vi "Drive_AutoShift (1).vi"(5 "Max":dbl format="%#_13g", 6 "Force Low Gear":bool, 7 "ShifterRef":T2={"DevStatus"={"status"=FALSE, "code"=0, "source"=""}, "Pneumatics Control Module"=0, "Forward Solenoid Channel"=enum."Invalid", "Reverse Solenoid Channel"=enum."Invalid"}, 8 "Right  Input":dbl, 9 "Left Input":dbl, 10 "Right RPM":dbl, 11 "Left RPM":dbl) -> (1 "Shifting":bool, 2 "Right Output":dbl, 3 "Left Output":dbl, 4 "Gear":T1)   [LabVIEW 2017]
uses:
  <vilib>/Rock Robotics/WPI/Solenoid/WPI_SolenoidDevRef.ctl
  <vilib>/Rock Robotics/WPI/Solenoid/WPI_SolenoidChannel.ctl
  <vilib>/Rock Robotics/WPI/Solenoid/WPI_SolenoidValue.ctl
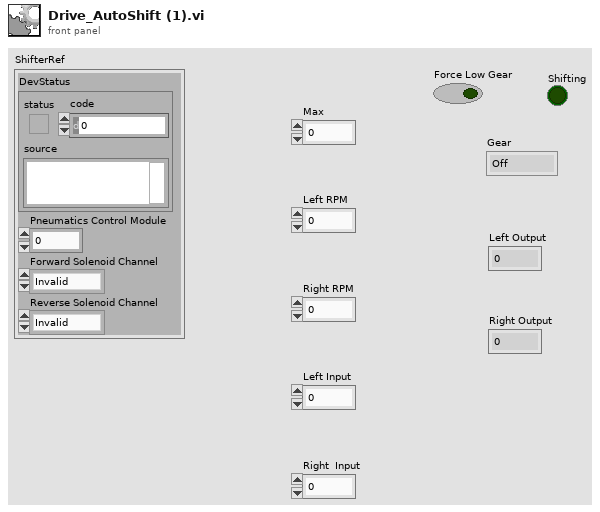
[diagram p1: front panel]
types:
  T1 = typedef "WPI_SolenoidValue.ctl" = enum16{"Off", "On", "Forward", "Reverse"}
  T2 = typedef "WPI_SolenoidDevRef.ctl" = cluster{"DevStatus":errorcluster, "Pneumatics Control Module":u8, "Forward Solenoid Channel":T3, "Reverse Solenoid Channel":T3}
  T3 = typedef "WPI_SolenoidChannel.ctl" = enum8{"Solenoid 0", "Solenoid 1", "Solenoid 2", "Solenoid 3", "Solenoid 4", "Solenoid 5", "Solenoid 6", "Solenoid 7", "Invalid"}
  T4 = cluster{"OutputMAX":dbl, "OutputMIN":dbl, "InputMAX":dbl, "InputMIN":dbl}
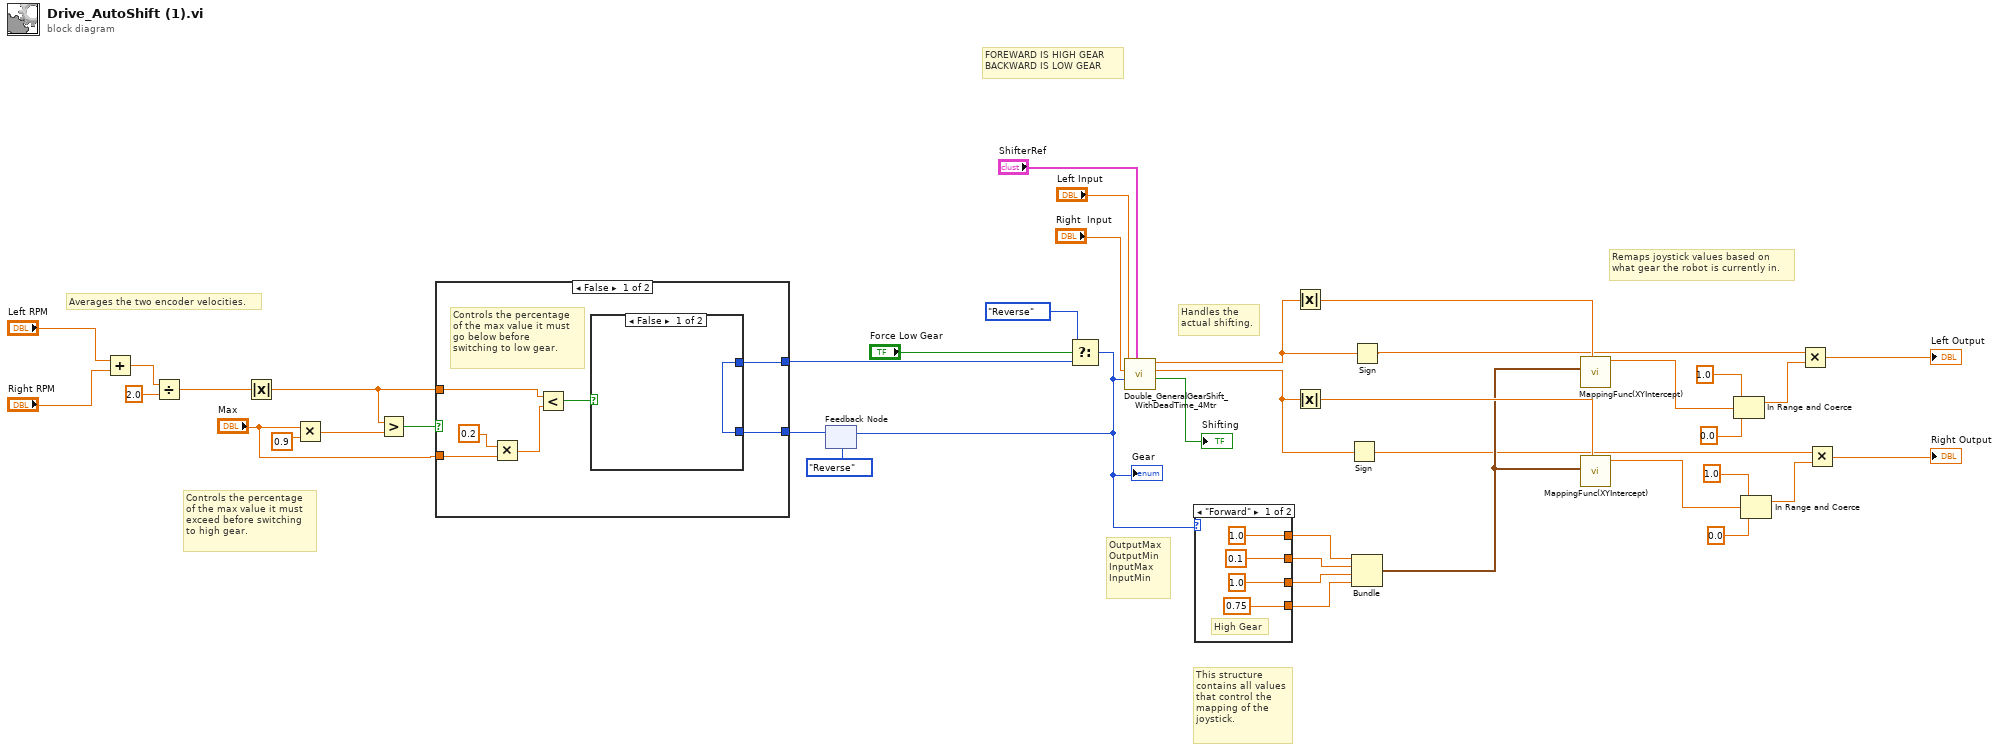
[diagram p0: block diagram]
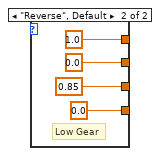
[diagram p2: hidden frame]
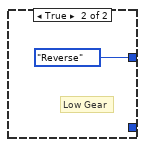
[diagram p3: hidden frame]
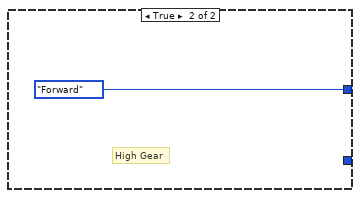
[diagram p4: hidden frame]
diagram:
  # "OutputMax\nOutputMin\nInputMax\nInputMin"
  # "This structure\ncontains all values\nthat control the\nmapping of the \njoystick."
  # "Remaps joystick values based on\nwhat gear the robot is currently in."
  # "Handles the\nactual shifting."
  # "FOREWARD IS HIGH GEAR\nBACKWARD IS LOW GEAR"
  # "Controls the percentage\nof the max value it must \nexceed before switching\nto high gear."
  # "Averages the two encoder velocities."
  n1 = Add(x="Left RPM", y="Right RPM") -> (x+y=w32:dbl)
  n2 = Divide(x=w32, y=2.0) -> (x/y=w12:dbl)
  n3 = Absolute Value(x=w12) -> (abs(x)=w11:dbl)
  n4 = Multiply(x="Max", y=0.9) -> (x*y=w40:dbl)
  n5 = Greater?(x=w11, y=w40) -> (0:w39:bool)
  n6 = feedback #1(WPI_SolenoidValue."Reverse" ("Shift Value")) -> (w9:T1)
  n7 = case shown="False" w39 {
    tunnel: [w44 WPI_SolenoidValue."Forward" ("Shift Value")] -> w23
    tunnel: "Max" -> [w47 _]
    tunnel: w9 -> [w43 _]
    tunnel: w11 -> [w42 _]
    frame False {
      # "Controls the percentage\nof the max value it must \ngo below before \nswitching to low gear."
      n8 = Multiply(x=0.2, y=w47) -> (x*y=w45:dbl)
      n9 = Less?(x=w42, y=w45) -> (x < y?=w48:bool)
      n10 = case shown="False" w48 {
        tunnel: [w49 WPI_SolenoidValue."Reverse" ("Shift Value")] -> w44
        tunnel: w43 -> [w49 _]
        frame False {
        }
        frame True {
          # "Low Gear"
        }
      }
    }
    frame True {
      # "High Gear"
    }
  }
  n11 = Select(t=WPI_SolenoidValue."Reverse", s="Force Low Gear", f=w23) -> (s? t:f=w1:T1)
  "Gear" <- w1
  n12 = feedback-in #1(w1) -> ()
  n13 = call "Double_GeneralGearShift_WithDeadTime_4Mtr.vi"("ShifterRef"="ShifterRef", "Shift Value"=w1, "Right"="Right  Input", "Left"="Left Input") -> ("Shifting"=→"Shifting":bool, "Right Output"=w6:dbl, "Left Output"=w7:dbl)  [unwired: 4 in, 1 out]
  n14 = case shown="\"Forward\"" w1 {
    tunnel: [1.0 ("OutputMAX") 1.0 ("OutputMAX")] -> w20
    tunnel: [0.1 ("OutputMIN") 0.0 ("OutputMIN")] -> w19
    tunnel: [1.0 ("InputMAX") 0.85 ("InputMAX")] -> w21
    tunnel: [0.75 ("InputMIN") 0.0 ("InputMIN")] -> w22
    frame "Forward" {
      # "High Gear"
    }
    frame "Reverse", Default {
      # "Low Gear"
    }
  }
  n15 = Absolute Value(x=w7) -> (abs(x)=w37:dbl)
  n16 = Absolute Value(x=w6) -> (abs(x)=w27:dbl)
  n17 = Sign(1:w6) -> (0:w17:dbl)
  n18 = Sign(1:w7) -> (0:w16:dbl)
  n19 = Bundle("OutputMAX"=w20, "OutputMIN"=w19, "InputMAX"=w21, "InputMIN"=w22) -> (w18:T4)  [unwired: 1 in]
  n20 = call "MappingFunc(XYIntercept).vi"("Input"=w37, "Cluster"=w18) -> ("Output"=w36:dbl)  [unwired: 9 in]
  n21 = call "MappingFunc(XYIntercept).vi"("Input"=w27, "Cluster"=w18) -> ("Output"=w28:dbl)  [unwired: 9 in]
  n22 = In Range and Coerce(upper limit=1.0, x=w36, lower limit=0.0) -> (coerced(x)=w33:dbl)  [unwired: 1 out]
  n23 = In Range and Coerce(upper limit=1.0, x=w28, lower limit=0.0) -> (coerced(x)=w29:dbl)  [unwired: 1 out]
  n24 = Multiply(x=w16, y=w33) -> (x*y=→"Left Output":dbl)
  n25 = Multiply(x=w17, y=w29) -> (x*y=→"Right Output":dbl)
